vi "digital_demod_host_sp_step.vi"() -> ()   [LabVIEW 2018]
uses:
  <vilib>/userdefined/High Color/nirio_resource_hc.ctl
  <vilib>/LabVIEW Targets/FPGA/RIO/nirio_PxiTriggers.ctl
  <vilib>/UPVI/lvhdf5/file.llb/LVH5F Operation.ctl
  <vilib>/UPVI/lvhdf5/dataset.llb/LVH5D Operation.ctl
  <vilib>/Utility/miscctls.llb/LVRectTypeDef.ctl
  <vilib>/UPVI/lvhdf5/group.llb/H5G_obj_t.ctl
  <vilib>/FPGAPlugInAG/PXI-7854R/niLvFpga_Open_PXI-7854R.vi
  <vilib>/rvi/interface/common/dynamic/niFpgaDynamicAddResources.vi
  <vilib>/FPGAPlugInAG/Dynamic/niLvFpga_Run_Dynamic.vi
  <vilib>/LabVIEW Targets/FPGA/RIO/nirioReserveTrigger.vi
  <vilib>/Utility/error.llb/Error Cluster From Error Code.vi
  <vilib>/rvi/errors/niLvFpgaAdjustHostInterfaceError.vi
  <vilib>/UPVI/lvhdf5/utility.llb/Select HDF5 Dialog.vi
  <vilib>/UPVI/lvhdf5/utility.llb/Select HDF5 Dialog (Object Only).vi
  <vilib>/UPVI/lvhdf5/dataset.llb/Simple H5Dwrite (Variant).vi
  <vilib>/FPGAPlugInAG/Dynamic/niLvFpga_Close_Dynamic.vi
  <vilib>/rvi/interface/nirviOpenFPGA/nirviOpenFPGA.xnode
  FPGA Bitfiles/digitaldemod_FPGATarget_digitaldemodfpga_GFAocKRMO-I.lvbitx
  <vilib>/rvi/interface/nirviMethod/nirviMethod.xnode
  <vilib>/rvi/interface/nirviReadWriteControl/nirviReadWriteControl.xnode
  <vilib>/UPVI/lvhdf5/dataset.llb/Simple H5Dwrite.xnode
  <vilib>/UPVI/lvhdf5/library.llb/HDF5 Ref.ctl
  <vilib>/rvi/interface/nirviCloseFPGA/nirviCloseFPGA.xnode
  <vilib>/rvi/interface/Simulation/niFpgaSimulationCallBeginRW.vi
  <vilib>/rvi/errors/niLvFpgaMergeErrorWithErrorCode.vi
  <vilib>/FPGAPlugInAG/Dynamic/niLvFpga_ReadFifo_Dynamic.vi
  NiFpgaLv.dll
  <vilib>/FPGAPlugInAG/Dynamic/niLvFpga_StartFifo_Dynamic.vi
  <vilib>/FPGAPlugInAG/Dynamic/niLvFpga_StopFifo_Dynamic.vi
  FPGA Timekeeper 1.1b0/FPGA Timekeeper.lvlib
  <vilib>/UPVI/lvhdf5/identifier.llb/Not an HDF5 Refnum Constant.vi
  <vilib>/UPVI/lvhdf5/dataset.llb/OpenCreateReplace Dataset by Element Type.vi
  <vilib>/UPVI/lvhdf5/dataspace.llb/H5Sselect_hyperslab.vi
  <vilib>/UPVI/lvhdf5/dataset.llb/H5Dwrite (Variant).vi
  <vilib>/UPVI/lvhdf5/dataset.llb/H5Dget_space.vi
  <vilib>/UPVI/lvhdf5/attribute.llb/private/LVH5AwriteWDTAttrs.vi
  <vilib>/UPVI/lvhdf5/dataspace.llb/H5Sclose.vi
  <vilib>/UPVI/lvhdf5/dataset.llb/H5Dclose.vi
  <vilib>/UPVI/lvhdf5/utility.llb/Select HDF5 Dialog (File and Object).vi
panel:
  in  "subtract_zfb_ndelay":u8=1
  in  "subtract_zfb_delay":bool=TRUE
  out "pow_fb":i16(graph)=-2000
  in  "subtract_zfb_i_scale":fxp<+/-,32,16>=-17.0
  in  "subtract_zfb_p_scale":fxp<+/-,32,16>=-23.0
  in  "subtract_zfb_d_scale":fxp<+/-,32,16>=-13.0
  in  "subtract_zfb_from_powerr":bool=TRUE
  in  "sum_z-pow_fb":bool=TRUE
  in  "delta_pow_set_llim":fxp<+/-,32,32>=-80000.0
  in  "delta_pow_set_ulim":fxp<+/-,32,32>=80000.0
  in  "fb_on_powset":bool
  in  "pow_lower_lim":i16=-2000
  in  "pow_upper_lim":i16=2000
  in  "pow_dc_offset":i16=-16000
  in  "pow_dg":fxp<+/-,32,16>
  in  "pow_pg":fxp<+/-,32,16>
  in  "pow_fb":bool=TRUE
  out "pow_set_actual":fxp<+/-,33,33>=-165000.0
  in  "reset_pow_accum":bool
  in  "pow_bitshift":i16=-6
  in  "pow_fb_bitshift":i16=-16
  in  "pow_ig":fxp<+/-,32,16>=0.001495361328125
  in  "pow_set_user":fxp<+/-,32,32>=-165000.0
  out "pow":i32(graph)=-95038
  out "delta_pow_set":dbl(graph)
  in  "DAQ_trig":bool
  in  "save_data":bool=TRUE
  out "z_fb_tot":i16(graph)=-20670
  in  "z_off_restart":bool
  in  "z_off_step":i16=-17500
  in  "z_off_start":i16=-17500
  in  "step_z_offset":bool
  in  "z_set_step":fxp<+/-,32,32>
  in  "step_z_set":bool
  out "z_set_user":fxp<+/-,32,32>
  in  "set_z_init":bool
  in  "reset_zphi_and_change":bool
  in  "reset_z_accum":bool
  in  "z_lower_lim":i16=-3000
  in  "z_upper_lim":i16=3000
  in  "z_fb_bitshift":i16=-16
  in  "z_ig":fxp<+/-,32,16>=-1.52587890625e-05
  in  "z_dg":fxp<+/-,32,16>=-0.100006103515625
  in  "z_pg":fxp<+/-,32,16>=-0.0200042724609375
  in  "z_bitshift":i16
  in  "z_set_init":fxp<+/-,32,32>
  in  "z_dc_offset":i16
  in  "z_internal_inject_scale":i16=400
  in  "z_internal_inject_freq":fxp<+,32,0>=2.00001522898674e-05 format="%#_32g"
  in  "add_sin":bool
  in  "show_quad":bool=TRUE
  out "delta_phi":cluster{dbl, dbl, dbl, dbl}(graph)={0.0, -13274.154479980469, -0.0958251953125, -57742.00476074219}
  in  "xy2_bitshift":i16
  in  "xy_fb_bitshift":i16=-16
  in  "y_lower_lim":i16=-1000
  in  "y_upper_lim":i16=1000
  in  "y_dg":fxp<+/-,32,16>=-0.0050048828125
  in  "x_lower_lim":i16=-1000
  in  "x_upper_lim":i16=1000
  in  "x_dg":fxp<+/-,32,16>=0.0050048828125
  in  "xy_bitshift":i16=-10
  in  "y_dc_offset":i16
  in  "x_dc_offset":i16
  in  "downsample->xyz":bool
  in  "inject_sigs":bool
  in  "Load last pars":bool
  out "config_trig":bool
  in  "block_hardware_trigs":bool
  out "config_loaded":bool
  out "Nsamp_config":u32=100000
  out "fpga_dat_path":path=path "D:/data/20201106/bead1/discharge/fine/turbombar_powfb_xyzcool_elec3_4000mV41Hz0mVdc_113_fpga.h5"
  in  "reset_trigs":bool
  in  "accept_trigs":bool=TRUE
  out "amp4":dbl(graph)=1195.7528991699219
  out "phi4":dbl(graph)=-7818.824462890625
  in  "Change Pars 2":bool
  out "z_fb":i16(graph)=-2670
  out "z":i32(graph)=-100000803
  out "y_fb":i16(graph)=-99
  out "y":i32(graph)=-476679
  out "x_fb":i16(graph)=-48
  out "x":i32(graph)=-117629
  out "Host time (ns)":u64=1605214259796328960
  out "Target time (ns)":u64=1605214259796293720
  in  "downsamp_num":i16=100
  in  "Reset Phi Params":T1={"All Phi?"=FALSE, "Which?"=enum."1"}
  out "amp2":dbl(graph)=13832.032684326172
  out "amp3":dbl(graph)=20215.12060546875
  out "amp0":dbl(graph)=9116.836563110352
  out "amp1":dbl(graph)=20779.648162841797
  out "phi2":dbl(graph)=-204.17840576171875
  out "phi3":dbl(graph)=-57946.087341308594
  in  "subtract_mean":bool=TRUE
  out "loop time":fxp<+,32,32>=2.0
  in  "Change Pars":bool
  out "phi0":dbl(graph)=-204.08258056640625
  out "phi1":dbl(graph)=-13478.237060546875
  in  "counter offset":u32
  in  "phase discont_neg":fxp<+/-,24,12>=-1.0
  in  "phase discont_pos":fxp<+/-,24,12>=1.0
  in  "Reset Phi":bool
  in  "loop timer (usec)":u32=2
  in  "Update ADC Clock":bool
  in  "Host Update Rate (msec)":dbl=1.0 format="%#_13g"
  in  "RIO Device":T2="RIO0"
  # "QPD AMPLITUDES"
  # "QPD PHASES"
  # "BACKSCATTER"
  # "BEAD XYZ + FB"
  # "FEEDBACK NESTING"
  # "POWER FEEDBACK"
  # "Z FEEDBACK"
  # "X FEEDBACK"
  # "Y FEEDBACK"
types:
  T1 = cluster{"All Phi?":bool, "Which?":enum16{"0", "1", "2", "3", "4"}}
  T2 = typedef "nirio_resource_hc.ctl" = tag
  T3 = typedef "nirio_PxiTriggers.ctl" = u16
  T4 = cluster{"phase discont_pos":fxp<+/-,24,12>, "phase discont_neg":fxp<+/-,24,12>, "counter offset":u32, "subtract_mean":bool, "downsamp_num":i16, "xy_bitshift":i16, "x_dg":fxp<+/-,32,16>, "x_upper_lim":i16, "x_lower_lim":i16, "x_dc_offset":i16, "y_dg":fxp<+/-,32,16>, "y_upper_lim":i16, "y_lower_lim":i16, "y_dc_offset":i16, "xy_fb_bitshift":i16, "z_bitshift":i16, "z_set_init":fxp<+/-,32,32>, "z_pg":fxp<+/-,32,16>, "z_dg":fxp<+/-,32,16>, "z_ig":fxp<+/-,32,16>, "z_fb_bitshift":i16, "z_upper_lim":i16, "z_lower_lim":i16, "z_off_start":i16, "inject_sigs":bool, "downsample->xyz":bool, "xy2_bitshift":i16, "add_sin":bool, "z_internal_inject_freq":fxp<+,32,0>, "z_internal_inject_scale":i16, "pow_bitshift":i16, "pow_set_user":fxp<+/-,32,32>, "pow_pg":fxp<+/-,32,16>, "pow_dg":fxp<+/-,32,16>, "pow_ig":fxp<+/-,32,16>, "pow_dc_offset":i16, "pow_upper_lim":i16, "pow_lower_lim":i16, "pow_fb_bitshift":i16, "pow_fb":bool, "fb_on_powset":bool, "delta_pow_set_ulim":fxp<+/-,32,32>, "delta_pow_set_llim":fxp<+/-,32,32>, "sum_z-pow_fb":bool, "subtract_zfb_from_powerr":bool, "subtract_zfb_p_scale":fxp<+/-,32,16>, "subtract_zfb_i_scale":fxp<+/-,32,16>, "subtract_zfb_d_scale":fxp<+/-,32,16>, "subtract_zfb_delay":bool, "subtract_zfb_ndelay":u8}
  T5 = enum16{"open", "replace", "create", "open or create", "replace or create", "replace or create with confirmation"}
  T6 = typedef "LVH5F Operation.ctl" = enum16{"open", "open or create", "create or replace", "create or replace (with confirmation)", "create", "open (read only)"}
  T7 = typedef "LVRectTypeDef.ctl" = cluster{"Left":i16, "Top":i16, "Right":i16, "Bottom":i16}
  T8 = cluster{"Behavior":enum32{"Invalid", "Default", "Floating", "Floating/Auto-Hide", "Modal"}, "Position":T7, "Center":bool, "Title":string}
  T9 = typedef "LVH5D Operation.ctl" = enum16{"open", "replace", "create", "open or create", "create or replace", "create or replace with confirmation"}
  T10 = typedef "H5G_obj_t.ctl" = i32
  T11 = cluster{"Object Types (any)":T10[], "Object Pattern":string}
  T12 = typedef "HDF5 Ref.ctl" = refnum<k1>
  T13 = cluster{fxp<+/-,33,19>, fxp<+/-,33,19>, fxp<+/-,33,19>, fxp<+/-,33,19>}
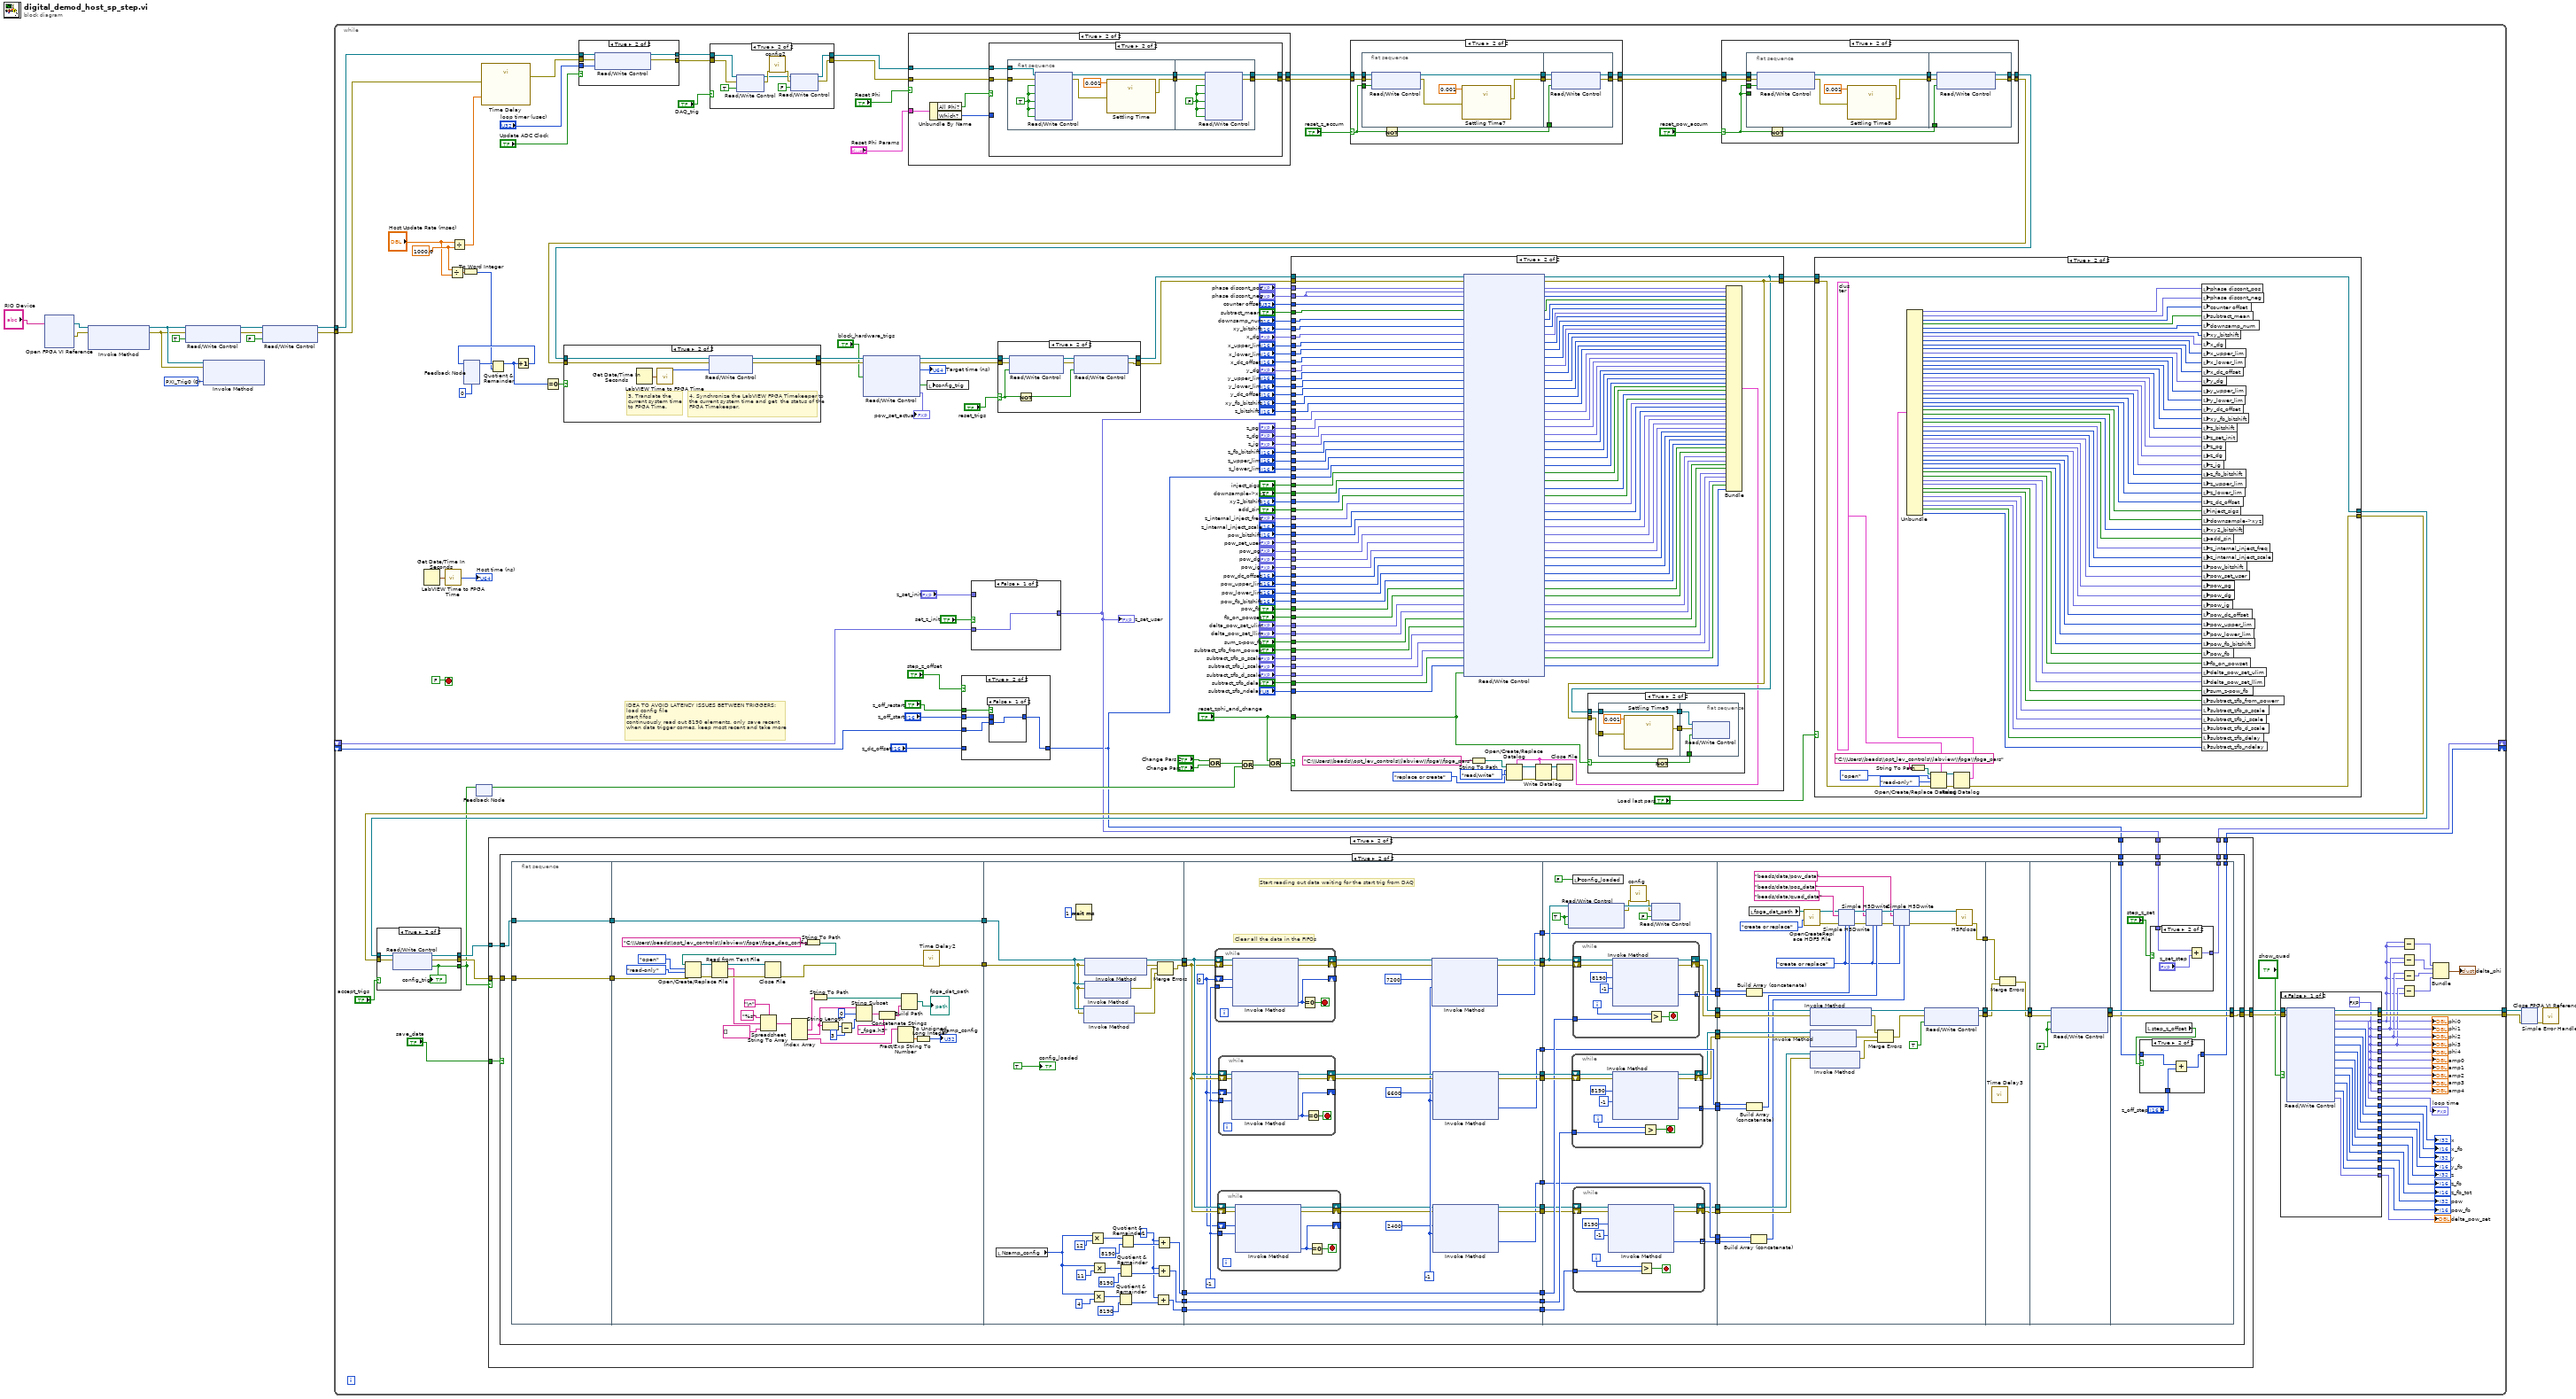
[diagram p0: block diagram]
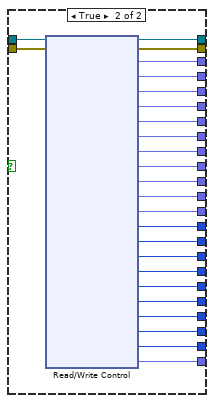
[diagram p7: hidden frame]
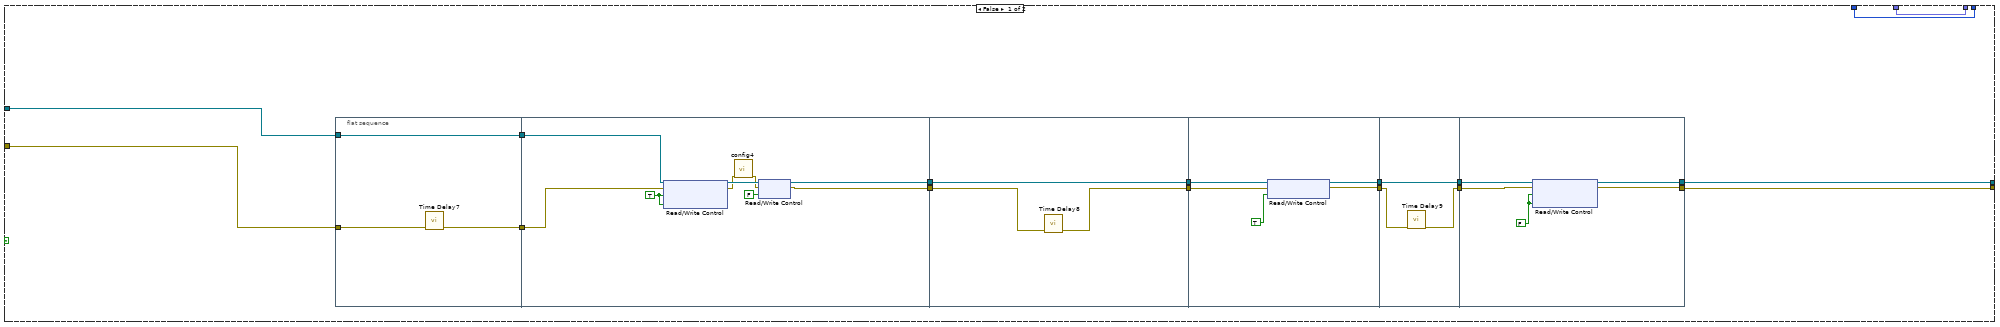
[diagram p12: hidden frame]
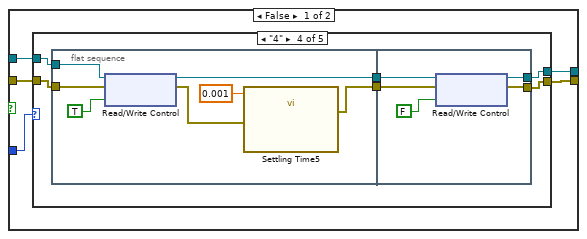
[diagram p20: hidden frame]
diagram:
  w1 = T3 0 items=["PXI_Trig0", "PXI_Trig1", "PXI_Trig2", "PXI_Trig3", "PXI_Trig4", "PXI_Trig5", "PXI_Trig6", "PXI_Trig7"] ("Trigger")
  n1 = xnode "Open FPGA VI Reference"("resource name"="RIO Device") -> ("FPGA VI Reference Out"=w11:refnum<k20>, "error out"=w10:errorcluster)  [unwired: 1 in]
  n2 = xnode "Invoke Method"("FPGA VI Reference In"=w11, "error in"=w10) -> ("FPGA VI Reference Out"=w3:refnum<k20>, "error out"=w2:errorcluster)  [unwired: 1 in]
  n3 = xnode "Read/Write Control"("FPGA VI Reference In"=w3, "error in"=w2, "reset_config_trig"=TRUE ("reset_trig")) -> ("FPGA VI Reference Out"=w6:refnum<k20>, "error out"=w4:errorcluster)
  n4 = xnode "Invoke Method"("FPGA VI Reference In"=w3, "error in"=w2, "Trigger"=w1) -> ()  [unwired: 2 out]
  n5 = xnode "Read/Write Control"("FPGA VI Reference In"=w6, "error in"=w4, "reset_config_trig"=FALSE ("manual_trig")) -> ("FPGA VI Reference Out"=w9:refnum<k20>, "error out"=w8:errorcluster)
  n6 = while {
    tunnel: w8 -> [w166]
    tunnel: w9 -> [w92]
    tunnel: [w159] -> w14
    tunnel: [w158] -> w13
    shift-right: [w70] -> _
    shift-left: _ -> [w71]
    shift-right: [w62] -> _
    shift-left: _ -> [w61]
    stop <- FALSE stop-if-true
    w149 = 1000.0
    # "IDEA TO AVOID LATENCY ISSUES BETWEEN TRIGGERS:\nload config file\nstart fifos\ncontinuously read out 8190 elements, only save recent\nwhen data trigger comes, keep most recent and take more"
    n7 = Get Date/Time In Seconds() -> (seconds since 1Jan1904=w138:timestamp)
    n8 = call "LabVIEW Time to FPGA Time.vi"("LabVIEW time"=w138) -> ("FPGA time (ns)"=→"Host time (ns)":u64)
    n9 = Divide(x=w149, y="Host Update Rate (msec)") -> (x/y=w147:dbl)
    n10 = Divide(x="Host Update Rate (msec)", y=w149) -> (x/y=w167:dbl)
    n11 = To Word Integer(number=w147) -> (16bit integer=w141:i16)
    n12 = feedback #1(i16 0) -> (w143:i16)
    n13 = feedback #2() -> (w73:bool)  [unwired: 1 in]
    n14 = call "Time Delay"("error in (no error)"=w166, "Delay Time (s)"=w167) -> ("error out"=w164:errorcluster)  [unwired: 9 in]
    n15 = Quotient & Remainder(x=w143, y=w141) -> (x-y*floor(x/y)=w140:i16)  [unwired: 1 out]
    n16 = Increment(x=w140) -> (x+1=w142:i16)
    n17 = feedback-in #1(w142) -> ()
    n18 = Equal To 0?(x=w140) -> (x = 0?=w145:bool)
    n19 = case shown="True" "Update ADC Clock" {
      tunnel: w92 -> [w1505 w1510]
      tunnel: w164 -> [w1504 w1509]
      tunnel: [w1505 w1508] -> w50
      tunnel: [w1504 w1507] -> w49
      tunnel: "loop timer (usec)" -> [_ w1506]
      frame False {
      }
      frame True {
        n20 = xnode "Read/Write Control"("FPGA VI Reference In"=w1510, "error in"=w1509, "loop timer (usec)"=w1506) -> ("FPGA VI Reference Out"=w1508:refnum<k20>, "error out"=w1507:errorcluster)
      }
    }
    n21 = case shown="True" "DAQ_trig" {
      tunnel: w50 -> [w191 w195]
      tunnel: w49 -> [w190 w194]
      tunnel: [w191 w193] -> w48
      tunnel: [w190 w192] -> w47
      frame False {
      }
      frame True {
        n22 = xnode "Read/Write Control"("FPGA VI Reference In"=w195, "error in"=w194, "TRIG0"=TRUE) -> ("FPGA VI Reference Out"=w197:refnum<k20>, "error out"=w198:errorcluster)
        n23 = call "config2"("error in (no error)"=w198) -> ("error out"=w199:errorcluster)  [unwired: 10 in]
        n24 = xnode "Read/Write Control"("FPGA VI Reference In"=w197, "error in"=w199, "TRIG0"=FALSE) -> ("FPGA VI Reference Out"=w193:refnum<k20>, "error out"=w192:errorcluster)
      }
    }
    n25 = case shown="True" "Reset Phi" {
      tunnel: w48 -> [w1383 w1390]
      tunnel: w47 -> [w1382 w1389]
      tunnel: [w1383 w1387] -> w96
      tunnel: [w1382 w1388] -> w95
      tunnel: "Reset Phi Params" -> [_ w1386]
      frame False {
      }
      frame True {
        n26 = Unbundle By Name(w1386) -> ("All Phi?"=w1385:bool, "Which?"=w1384:enum16{"0", "1", "2", "3", "4"})
        n27 = case shown="True" w1385 {
          tunnel: w1390 -> [w1395 w1489]
          tunnel: w1389 -> [w1394 w1488]
          tunnel: [w1392 w1487] -> w1388
          tunnel: [w1393 w1486] -> w1387
          tunnel: w1384 -> [w1391 _]
          frame False {
            n28 = case shown="\"4\"" w1391 {
              tunnel: w1395 -> [w1399 w1417 w1435 w1453 w1471]
              tunnel: w1394 -> [w1398 w1416 w1434 w1452 w1470]
              tunnel: [w1397 w1415 w1433 w1451 w1469] -> w1393
              tunnel: [w1396 w1414 w1432 w1450 w1468] -> w1392
              frame "1" {
                n29 = flat-sequence {
                  tunnel: w1399 -> [w1408]
                  tunnel: w1398 -> [w1407]
                  tunnel: [w1406] -> w1401
                  tunnel: [w1403] -> w1400
                  tunnel: w1401 -> [w1413]
                  tunnel: w1400 -> [w1412]
                  tunnel: [w1411] -> w1397
                  tunnel: [w1410] -> w1396
                  frame #0 {
                    n30 = xnode "Read/Write Control"("FPGA VI Reference In"=w1408, "error in"=w1407, "reset_phi1"=TRUE) -> ("FPGA VI Reference Out"=w1406:refnum<k20>, "error out"=w1404:errorcluster)
                    n31 = call "Settling Time2"("error in (no error)"=w1404, "Delay Time (s)"=0.001) -> ("error out"=w1403:errorcluster)  [unwired: 9 in]
                  }
                  frame #1 {
                    n32 = xnode "Read/Write Control"("FPGA VI Reference In"=w1413, "error in"=w1412, "reset_phi1"=FALSE) -> ("FPGA VI Reference Out"=w1411:refnum<k20>, "error out"=w1410:errorcluster)
                  }
                }
              }
              frame "2" {
                n33 = flat-sequence {
                  tunnel: w1417 -> [w1426]
                  tunnel: w1416 -> [w1425]
                  tunnel: [w1424] -> w1419
                  tunnel: [w1421] -> w1418
                  tunnel: w1419 -> [w1431]
                  tunnel: w1418 -> [w1430]
                  tunnel: [w1429] -> w1415
                  tunnel: [w1428] -> w1414
                  frame #0 {
                    n34 = xnode "Read/Write Control"("FPGA VI Reference In"=w1426, "error in"=w1425, "reset_phi2"=TRUE) -> ("FPGA VI Reference Out"=w1424:refnum<k20>, "error out"=w1422:errorcluster)
                    n35 = call "Settling Time3"("error in (no error)"=w1422, "Delay Time (s)"=0.001) -> ("error out"=w1421:errorcluster)  [unwired: 9 in]
                  }
                  frame #1 {
                    n36 = xnode "Read/Write Control"("FPGA VI Reference In"=w1431, "error in"=w1430, "reset_phi2"=FALSE) -> ("FPGA VI Reference Out"=w1429:refnum<k20>, "error out"=w1428:errorcluster)
                  }
                }
              }
              frame "3" {
                n37 = flat-sequence {
                  tunnel: w1435 -> [w1444]
                  tunnel: w1434 -> [w1443]
                  tunnel: [w1442] -> w1437
                  tunnel: [w1439] -> w1436
                  tunnel: w1437 -> [w1449]
                  tunnel: w1436 -> [w1448]
                  tunnel: [w1447] -> w1433
                  tunnel: [w1446] -> w1432
                  frame #0 {
                    n38 = xnode "Read/Write Control"("FPGA VI Reference In"=w1444, "error in"=w1443, "reset_phi3"=TRUE) -> ("FPGA VI Reference Out"=w1442:refnum<k20>, "error out"=w1440:errorcluster)
                    n39 = call "Settling Time4"("error in (no error)"=w1440, "Delay Time (s)"=0.001) -> ("error out"=w1439:errorcluster)  [unwired: 9 in]
                  }
                  frame #1 {
                    n40 = xnode "Read/Write Control"("FPGA VI Reference In"=w1449, "error in"=w1448, "reset_phi3"=FALSE) -> ("FPGA VI Reference Out"=w1447:refnum<k20>, "error out"=w1446:errorcluster)
                  }
                }
              }
              frame "4" {
                n41 = flat-sequence {
                  tunnel: w1453 -> [w1462]
                  tunnel: w1452 -> [w1461]
                  tunnel: [w1460] -> w1455
                  tunnel: [w1457] -> w1454
                  tunnel: w1455 -> [w1467]
                  tunnel: w1454 -> [w1466]
                  tunnel: [w1465] -> w1451
                  tunnel: [w1464] -> w1450
                  frame #0 {
                    n42 = xnode "Read/Write Control"("FPGA VI Reference In"=w1462, "error in"=w1461, "reset_phi4"=TRUE) -> ("FPGA VI Reference Out"=w1460:refnum<k20>, "error out"=w1458:errorcluster)
                    n43 = call "Settling Time5"("error in (no error)"=w1458, "Delay Time (s)"=0.001) -> ("error out"=w1457:errorcluster)  [unwired: 9 in]
                  }
                  frame #1 {
                    n44 = xnode "Read/Write Control"("FPGA VI Reference In"=w1467, "error in"=w1466, "reset_phi4"=FALSE) -> ("FPGA VI Reference Out"=w1465:refnum<k20>, "error out"=w1464:errorcluster)
                  }
                }
              }
              frame "0" {
                n45 = flat-sequence {
                  tunnel: w1471 -> [w1480]
                  tunnel: w1470 -> [w1479]
                  tunnel: [w1478] -> w1473
                  tunnel: [w1475] -> w1472
                  tunnel: w1473 -> [w1485]
                  tunnel: w1472 -> [w1484]
                  tunnel: [w1483] -> w1469
                  tunnel: [w1482] -> w1468
                  frame #0 {
                    n46 = xnode "Read/Write Control"("FPGA VI Reference In"=w1480, "error in"=w1479, "reset_phi0"=TRUE) -> ("FPGA VI Reference Out"=w1478:refnum<k20>, "error out"=w1476:errorcluster)
                    n47 = call "Settling Time6"("error in (no error)"=w1476, "Delay Time (s)"=0.001) -> ("error out"=w1475:errorcluster)  [unwired: 9 in]
                  }
                  frame #1 {
                    n48 = xnode "Read/Write Control"("FPGA VI Reference In"=w1485, "error in"=w1484, "reset_phi0"=FALSE) -> ("FPGA VI Reference Out"=w1483:refnum<k20>, "error out"=w1482:errorcluster)
                  }
                }
              }
            }
          }
          frame True {
            n49 = flat-sequence {
              tunnel: w1489 -> [w1498]
              tunnel: w1488 -> [w1497]
              tunnel: [w1496] -> w1491
              tunnel: [w1493] -> w1490
              tunnel: w1491 -> [w1503]
              tunnel: w1490 -> [w1502]
              tunnel: [w1501] -> w1486
              tunnel: [w1500] -> w1487
              frame #0 {
                w1492 = TRUE
                n50 = xnode "Read/Write Control"("FPGA VI Reference In"=w1498, "error in"=w1497, "reset_phi0"=w1492, "reset_phi1"=w1492, "reset_phi2"=w1492, "reset_phi3"=w1492, "reset_phi4"=w1492) -> ("FPGA VI Reference Out"=w1496:refnum<k20>, "error out"=w1494:errorcluster)
                n51 = call "Settling Time"("error in (no error)"=w1494, "Delay Time (s)"=0.001) -> ("error out"=w1493:errorcluster)  [unwired: 9 in]
              }
              frame #1 {
                w1499 = FALSE
                n52 = xnode "Read/Write Control"("FPGA VI Reference In"=w1503, "error in"=w1502, "reset_phi0"=w1499, "reset_phi1"=w1499, "reset_phi2"=w1499, "reset_phi3"=w1499, "reset_phi4"=w1499) -> ("FPGA VI Reference Out"=w1501:refnum<k20>, "error out"=w1500:errorcluster)
              }
            }
          }
        }
      }
    }
    n53 = case shown="True" "step_z_offset" {
      tunnel: [w201 w202] -> w63
      tunnel: "z_dc_offset" -> [w201 _]
      tunnel: w61 -> [_ w204]
      tunnel: "z_off_start" -> [_ w205]
      tunnel: "z_off_restart" -> [_ w203]
      frame False {
      }
      frame True {
        n54 = case shown="False" w203 {
          tunnel: w205 -> [_ w207]
          tunnel: w204 -> [w206 _]
          tunnel: [w206 w207] -> w202
          frame False {
          }
          frame True {
          }
        }
      }
    }
    n55 = case shown="False" "set_z_init" {
      tunnel: [w208 w209] -> w69
      tunnel: "z_set_init" -> [_ w209]
      tunnel: w71 -> [w208 _]
      frame False {
      }
      frame True {
      }
    }
    "z_set_user" <- w69
    n56 = Or(x="Change Pars 2", y="Change Pars") -> (x .or. y?=w24:bool)
    n57 = Or(x=w24, y=w73) -> (x .or. y?=w22:bool)
    n58 = Or(x="reset_zphi_and_change", y=w22) -> (x .or. y?=w21:bool)
    n59 = case shown="True" "reset_z_accum" {
      selector: "reset_z_accum" -> [_ w317]
      tunnel: w96 -> [w315 w323]
      tunnel: w95 -> [w314 w322]
      tunnel: [w315 w321] -> w46
      tunnel: [w314 w320] -> w45
      frame False {
      }
      frame True {
        n60 = flat-sequence {
          tunnel: w323 -> [w330]
          tunnel: w322 -> [w329]
          tunnel: w317 -> [w327]
          tunnel: [w328] -> w319
          tunnel: [w324] -> w318
          tunnel: [w332] -> w320
          tunnel: [w333] -> w321
          tunnel: w319 -> [w335]
          tunnel: w318 -> [w334]
          tunnel: w316 -> [w331]
          frame #0 {
            n61 = xnode "Read/Write Control"("FPGA VI Reference In"=w330, "error in"=w329, "reset_z_accum"=w327) -> ("FPGA VI Reference Out"=w328:refnum<k20>, "error out"=w325:errorcluster)
            n62 = call "Settling Time7"("error in (no error)"=w325, "Delay Time (s)"=0.001) -> ("error out"=w324:errorcluster)  [unwired: 9 in]
          }
          frame #1 {
            n63 = xnode "Read/Write Control"("FPGA VI Reference In"=w335, "error in"=w334, "reset_z_accum"=w331) -> ("FPGA VI Reference Out"=w333:refnum<k20>, "error out"=w332:errorcluster)
          }
        }
        n64 = Not(x=w317) -> (.not. x?=w316:bool)
      }
    }
    n65 = case shown="True" "reset_pow_accum" {
      selector: "reset_pow_accum" -> [_ w172]
      tunnel: w46 -> [w169 w174]
      tunnel: w45 -> [w168 w173]
      tunnel: [w169 w171] -> w43
      tunnel: [w168 w170] -> w42
      frame False {
      }
      frame True {
        n66 = flat-sequence {
          tunnel: w174 -> [w184]
          tunnel: w173 -> [w183]
          tunnel: w172 -> [w181]
          tunnel: [w182] -> w177
          tunnel: [w178] -> w176
          tunnel: w172 -> [_]
          tunnel: [w185] -> _
          tunnel: [w187] -> w171
          tunnel: w177 -> [w189]
          tunnel: w176 -> [w188]
          tunnel: w175 -> [w186]
          tunnel: [w185] -> w170
          frame #0 {
            n67 = xnode "Read/Write Control"("FPGA VI Reference In"=w184, "error in"=w183, "reset_pow_accum"=w181) -> ("FPGA VI Reference Out"=w182:refnum<k20>, "error out"=w179:errorcluster)
            n68 = call "Settling Time8"("error in (no error)"=w179, "Delay Time (s)"=0.001) -> ("error out"=w178:errorcluster)  [unwired: 9 in]
          }
          frame #1 {
            n69 = xnode "Read/Write Control"("FPGA VI Reference In"=w189, "error in"=w188, "reset_pow_accum"=w186) -> ("FPGA VI Reference Out"=w187:refnum<k20>, "error out"=w185:errorcluster)
          }
        }
        n70 = Not(x=w172) -> (.not. x?=w175:bool)
      }
    }
    n71 = case shown="True" w145 {
      tunnel: w42 -> [w1295 w1300]
      tunnel: w43 -> [w1296 w1299]
      tunnel: [w1296 w1298] -> w136
      tunnel: [w1295 w1297] -> w135
      frame False {
      }
      frame True {
        # "4. Synchronize the LabVIEW FPGA Timekeeper to the current system time and get  the status of the FPGA Timekeeper."
        # "3. Translate the current system time to FPGA Time."
        n72 = Get Date/Time In Seconds() -> (seconds since 1Jan1904=w1302:timestamp)
        n73 = call "LabVIEW Time to FPGA Time.vi"("LabVIEW time"=w1302) -> ("FPGA time (ns)"=w1301:u64)
        n74 = xnode "Read/Write Control"("FPGA VI Reference In"=w1299, "error in"=w1300, "RT time (ns)"=w1301) -> ("FPGA VI Reference Out"=w1298:refnum<k20>, "error out"=w1297:errorcluster)
      }
    }
    n75 = xnode "Read/Write Control"("FPGA VI Reference In"=w136, "error in"=w135, "block_config_trig"="block_hardware_trigs") -> ("FPGA VI Reference Out"=w107:refnum<k20>, "error out"=w106:errorcluster, "time (ns)"=→"Target time (ns)":u64, "config_trig"=w93:bool, "pow_set_actual"=→"pow_set_actual":fxp<+/-,33,33>)
    n76 = local write "config_trig"(w93) -> ()
    n77 = case shown="True" "reset_trigs" {
      selector: "reset_trigs" -> [_ w1288]
      tunnel: w107 -> [w1286 w1294]
      tunnel: w106 -> [w1285 w1293]
      tunnel: [w1286 w1290] -> w103
      tunnel: [w1285 w1289] -> w102
      frame False {
      }
      frame True {
        n78 = xnode "Read/Write Control"("FPGA VI Reference In"=w1294, "error in"=w1293, "reset_config_trig"=w1288) -> ("FPGA VI Reference Out"=w1292:refnum<k20>, "error out"=w1291:errorcluster)
        n79 = Not(x=w1288) -> (.not. x?=w1287:bool)
        n80 = xnode "Read/Write Control"("FPGA VI Reference In"=w1292, "error in"=w1291, "reset_config_trig"=w1287) -> ("FPGA VI Reference Out"=w1290:refnum<k20>, "error out"=w1289:errorcluster)
      }
    }
    n81 = case shown="True" w21 {
      tunnel: w102 -> [w1304 w1367]
      tunnel: [w1304 w1310] -> w89
      tunnel: [w1303 w1309] -> w91
      tunnel: w103 -> [w1303 w1368]
      tunnel: "phase discont_pos" -> [_ w1366]
      tunnel: "phase discont_neg" -> [_ w1365]
      tunnel: "counter offset" -> [_ w1364]
      tunnel: "subtract_mean" -> [_ w1363]
      tunnel: "downsamp_num" -> [_ w1362]
      tunnel: "x_dc_offset" -> [_ w1357]
      tunnel: "y_dc_offset" -> [_ w1353]
      tunnel: w63 -> [_ w1343]
      tunnel: w69 -> [_ w1350]
      tunnel: "xy_bitshift" -> [_ w1361]
      tunnel: "x_dg" -> [_ w1360]
      tunnel: "x_upper_lim" -> [_ w1359]
      tunnel: "x_lower_lim" -> [_ w1358]
      tunnel: "y_dg" -> [_ w1356]
      tunnel: "y_upper_lim" -> [_ w1355]
      tunnel: "y_lower_lim" -> [_ w1354]
      tunnel: "z_bitshift" -> [_ w1351]
      tunnel: "z_pg" -> [_ w1349]
      tunnel: "z_dg" -> [_ w1348]
      tunnel: "z_ig" -> [_ w1347]
      tunnel: "z_fb_bitshift" -> [_ w1346]
      tunnel: "z_upper_lim" -> [_ w1345]
      tunnel: "z_lower_lim" -> [_ w1344]
      tunnel: "xy_fb_bitshift" -> [_ w1352]
      tunnel: "inject_sigs" -> [_ w1334]
      tunnel: "downsample->xyz" -> [_ w1333]
      tunnel: "xy2_bitshift" -> [_ w1332]
      tunnel: "add_sin" -> [_ w1331]
      tunnel: "z_internal_inject_freq" -> [_ w1330]
      tunnel: "z_internal_inject_scale" -> [_ w1329]
      tunnel: "pow_set_user" -> [_ w1327]
      tunnel: "pow_ig" -> [_ w1326]
      tunnel: "pow_fb_bitshift" -> [_ w1320]
      tunnel: "pow_bitshift" -> [_ w1328]
      tunnel: "fb_on_powset" -> [_ w1318]
      tunnel: "delta_pow_set_ulim" -> [_ w1317]
      tunnel: "delta_pow_set_llim" -> [_ w1316]
      tunnel: "pow_fb" -> [_ w1319]
      tunnel: "pow_pg" -> [_ w1324]
      tunnel: "pow_dg" -> [_ w1325]
      tunnel: "pow_dc_offset" -> [_ w1323]
      tunnel: "pow_upper_lim" -> [_ w1322]
      tunnel: "pow_lower_lim" -> [_ w1321]
      tunnel: "sum_z-pow_fb" -> [_ w1315]
      tunnel: "subtract_zfb_from_powerr" -> [_ w1314]
      tunnel: "subtract_zfb_d_scale" -> [_ w1313]
      tunnel: "subtract_zfb_p_scale" -> [_ w1312]
      tunnel: "subtract_zfb_i_scale" -> [_ w1311]
      tunnel: "reset_zphi_and_change" -> [_ w1307]
      tunnel: "subtract_zfb_delay" -> [_ w1306]
      tunnel: "subtract_zfb_ndelay" -> [_ w1305]
      frame False {
      }
      frame True {
        n82 = xnode "Read/Write Control"("FPGA VI Reference In"=w1368, "error in"=w1367, "discont_pos"=w1366, "discont_neg"=w1365, "Counter Offset"=w1364, "subtract_mean"=w1363, "downsamp_num"=w1362, "xy_bitshift"=w1361, "x_dg"=w1360, "x_upper_lim"=w1359, "x_lower_lim"=w1358, "x_dc_offset"=w1357, "y_dg"=w1356, "y_upper_lim"=w1355, "y_lower_lim"=w1354, "y_dc_offset"=w1353, "xy_fb_bitshift"=w1352, "z_bitshift"=w1351, "z_set_user"=w1350, "z_pg"=w1349, "z_dg"=w1348, "z_ig"=w1347, "z_fb_bitshift"=w1346, "z_upper_lim"=w1345, "z_lower_lim"=w1344, "z_dc_offset"=w1343, "inject_sigs"=w1334, "downsample->xyz"=w1333, "xy2_bitshift"=w1332, "add_sin"=w1331, "z_internal_inject_freq"=w1330, "z_internal_inject_scale"=w1329, "pow_bitshift"=w1328, "pow_set_user"=w1327, "pow_pg"=w1324, "pow_dg"=w1325, "pow_ig"=w1326, "pow_dc_offset"=w1323, "pow_upper_lim"=w1322, "pow_lower_lim"=w1321, "pow_fb_bitshift"=w1320, "pow_fb"=w1319, "fb_on_pow_set"=w1318, "delta_pow_set_ulim"=w1317, "delta_pow_set_llim"=w1316, "sum_z-pow_fb"=w1315, "subtract_zfb_from_powerr"=w1314, "subtract_zfb_p_scale"=w1312, "subtract_zfb_i_scale"=w1311, "subtract_zfb_d_scale"=w1313, "subtract_zfb_delay"=w1306, "subtract_zfb_ndelay"=w1305, "reset_phi4"=w1307) -> ("FPGA VI Reference Out"=w1309:refnum<k20>, "error out"=w1310:errorcluster)
        n83 = String To Path(string="C:\\Users\\beads\\opt_lev_controls\\labview\\fpga\\fpga_pars") -> (path=w1336:path)
        n84 = case shown="True" w1307 {
          selector: w1307 -> [_ w1370]
          tunnel: w1310 -> [_ w1372]
          tunnel: w1309 -> [_ w1373]
          frame False {
          }
          frame True {
            n85 = flat-sequence {
              tunnel: [w1377] -> w1374
              tunnel: w1373 -> [w1377]
              tunnel: w1372 -> [w1376]
              tunnel: [w1375] -> w1371
              tunnel: w1374 -> [w1381]
              tunnel: w1371 -> [w1380]
              tunnel: w1369 -> [w1379]
              frame #0 {
                n86 = call "Settling Time9"("error in (no error)"=w1376, "Delay Time (s)"=0.001) -> ("error out"=w1375:errorcluster)  [unwired: 9 in]
              }
              frame #1 {
                n87 = xnode "Read/Write Control"("FPGA VI Reference In"=w1381, "error in"=w1380, "reset_phi4"=w1379) -> ()  [unwired: 2 out]
              }
            }
            n88 = Not(x=w1370) -> (.not. x?=w1369:bool)
          }
        }
        n89 = Bundle("phase discont_pos"=w1366, "phase discont_neg"=w1365, "counter offset"=w1364, "subtract_mean"=w1363, "downsamp_num"=w1362, "xy_bitshift"=w1361, "x_dg"=w1360, "x_upper_lim"=w1359, "x_lower_lim"=w1358, "x_dc_offset"=w1357, "y_dg"=w1356, "y_upper_lim"=w1355, "y_lower_lim"=w1354, "y_dc_offset"=w1353, "xy_fb_bitshift"=w1352, "z_bitshift"=w1351, "z_set_init"=w1350, "z_pg"=w1349, "z_dg"=w1348, "z_ig"=w1347, "z_fb_bitshift"=w1346, "z_upper_lim"=w1345, "z_lower_lim"=w1344, "z_off_start"=w1343, "inject_sigs"=w1334, "downsample->xyz"=w1333, "xy2_bitshift"=w1332, "add_sin"=w1331, "z_internal_inject_freq"=w1330, "z_internal_inject_scale"=w1329, "pow_bitshift"=w1328, "pow_set_user"=w1327, "pow_pg"=w1324, "pow_dg"=w1325, "pow_ig"=w1326, "pow_dc_offset"=w1323, "pow_upper_lim"=w1322, "pow_lower_lim"=w1321, "pow_fb_bitshift"=w1320, "pow_fb"=w1319, "fb_on_powset"=w1318, "delta_pow_set_ulim"=w1317, "delta_pow_set_llim"=w1316, "sum_z-pow_fb"=w1315, "subtract_zfb_from_powerr"=w1314, "subtract_zfb_p_scale"=w1312, "subtract_zfb_i_scale"=w1311, "subtract_zfb_d_scale"=w1313, "subtract_zfb_delay"=w1306, "subtract_zfb_ndelay"=w1305) -> (w1308:T4)  [unwired: 1 in]
        n90 = Open/Create/Replace Datalog(5:w1308, 9:enum16{"read/write", "read-only", "write-only"}."read/write" ("access (0:read/write)"), 10:T5."replace or create" ("operation (0:open)"), 11:w1336) -> (0:w1342:errorcluster, 3:w1340:refnum<k1>)  [unwired: 2 in, 1 out]
        n91 = Write Datalog(4:w1342, 6:w1308, 7:w1340) -> (0:w1341:errorcluster, 3:w1339:refnum<k1>)
        n92 = Close File(refnum=w1339, error in=w1341) -> ()  [unwired: 2 out]
      }
    }
    n93 = case shown="True" "Load last pars" {
      tunnel: [w252 w309] -> w90
      tunnel: w91 -> [w252 w309]
      tunnel: [w251 w296] -> w88
      tunnel: w89 -> [w251 w310]
      frame False {
      }
      frame True {
        n94 = String To Path(string="C:\\Users\\beads\\opt_lev_controls\\labview\\fpga\\fpga_pars") -> (path=w313:path)
        n95 = Open/Create/Replace Datalog(5:T4 {"phase discont_pos"=0.0, "phase discont_neg"=0.0, "counter offset"=0, "subtract_mean"=FALSE, "downsamp_num"=0, "xy_bitshift"=0, "x_dg"=0.0, "x_upper_lim"=0, "x_lower_lim"=0, "x_dc_offset"=0, "y_dg"=0.0, "y_upper_lim"=0, "y_lower_lim"=0, "y_dc_offset"=0, "xy_fb_bitshift"=0, "z_bitshift"=0, "z_set_init"=0.0, "z_pg"=0.0, "z_dg"=0.0, "z_ig"=0.0, "z_fb_bitshift"=0, "z_upper_lim"=0, "z_lower_lim"=0, "z_off_start"=0, "inject_sigs"=FALSE, "downsample->xyz"=FALSE, "xy2_bitshift"=0, "add_sin"=FALSE, "z_internal_inject_freq"=0.0, "z_internal_inject_scale"=0, "pow_bitshift"=0, "pow_set_user"=0.0, "pow_pg"=0.0, "pow_dg"=0.0, "pow_ig"=0.0, "pow_dc_offset"=0, "pow_upper_lim"=0, "pow_lower_lim"=0, "pow_fb_bitshift"=0, "pow_fb"=FALSE, "fb_on_powset"=FALSE, "delta_pow_set_ulim"=0.0, "delta_pow_set_llim"=0.0, "sum_z-pow_fb"=FALSE, "subtract_zfb_from_powerr"=FALSE, "subtract_zfb_p_scale"=0.0, "subtract_zfb_i_scale"=0.0, "subtract_zfb_d_scale"=0.0, "subtract_zfb_delay"=FALSE, "subtract_zfb_ndelay"=0} ("output cluster"), 8:w310, 9:enum16{"read/write", "read-only", "write-only"}."read-only" ("access (0:read/write)"), 10:T5."open" ("operation (0:open)"), 11:w313) -> (0:w307:errorcluster, 3:w308:refnum<k1>)  [unwired: 1 in, 1 out]
        n96 = Read Datalog(4:w307, 7:w308) -> (0:w296:errorcluster, 2:w306:T4)  [unwired: 1 in, 1 out]
        n97 = Unbundle(w306) -> ("phase discont_pos"=w305:fxp<+/-,24,12>, "phase discont_neg"=w304:fxp<+/-,24,12>, "counter offset"=w303:u32, "subtract_mean"=w302:bool, "downsamp_num"=w301:i16, "xy_bitshift"=w300:i16, "x_dg"=w299:fxp<+/-,32,16>, "x_upper_lim"=w298:i16, "x_lower_lim"=w297:i16, "x_dc_offset"=w295:i16, "y_dg"=w294:fxp<+/-,32,16>, "y_upper_lim"=w293:i16, "y_lower_lim"=w292:i16, "y_dc_offset"=w291:i16, "xy_fb_bitshift"=w290:i16, "z_bitshift"=w289:i16, "z_set_init"=w288:fxp<+/-,32,32>, "z_pg"=w287:fxp<+/-,32,16>, "z_dg"=w286:fxp<+/-,32,16>, "z_ig"=w285:fxp<+/-,32,16>, "z_fb_bitshift"=w284:i16, "z_upper_lim"=w283:i16, "z_lower_lim"=w282:i16, "z_off_start"=w281:i16, "inject_sigs"=w279:bool, "downsample->xyz"=w278:bool, "xy2_bitshift"=w277:i16, "add_sin"=w276:bool, "z_internal_inject_freq"=w275:fxp<+,32,0>, "z_internal_inject_scale"=w274:i16, "pow_bitshift"=w273:i16, "pow_set_user"=w272:fxp<+/-,32,32>, "pow_pg"=w271:fxp<+/-,32,16>, "pow_dg"=w270:fxp<+/-,32,16>, "pow_ig"=w269:fxp<+/-,32,16>, "pow_dc_offset"=w268:i16, "pow_upper_lim"=w267:i16, "pow_lower_lim"=w266:i16, "pow_fb_bitshift"=w265:i16, "pow_fb"=w264:bool, "fb_on_powset"=w263:bool, "delta_pow_set_ulim"=w262:fxp<+/-,32,32>, "delta_pow_set_llim"=w261:fxp<+/-,32,32>, "sum_z-pow_fb"=w260:bool, "subtract_zfb_from_powerr"=w259:bool, "subtract_zfb_p_scale"=w258:fxp<+/-,32,16>, "subtract_zfb_i_scale"=w257:fxp<+/-,32,16>, "subtract_zfb_d_scale"=w256:fxp<+/-,32,16>, "subtract_zfb_delay"=w254:bool, "subtract_zfb_ndelay"=w253:u8)
        n98 = local write "phase discont_pos"(w305) -> ()
        n99 = local write "phase discont_neg"(w304) -> ()
        n100 = local write "counter offset"(w303) -> ()
        n101 = local write "subtract_mean"(w302) -> ()
        n102 = local write "downsamp_num"(w301) -> ()
        n103 = local write "xy_bitshift"(w300) -> ()
        n104 = local write "x_dg"(w299) -> ()
        n105 = local write "x_upper_lim"(w298) -> ()
        n106 = local write "x_lower_lim"(w297) -> ()
        n107 = local write "x_dc_offset"(w295) -> ()
        n108 = local write "y_dg"(w294) -> ()
        n109 = local write "y_upper_lim"(w293) -> ()
        n110 = local write "y_lower_lim"(w292) -> ()
        n111 = local write "y_dc_offset"(w291) -> ()
        n112 = local write "xy_fb_bitshift"(w290) -> ()
        n113 = local write "z_bitshift"(w289) -> ()
        n114 = local write "z_set_init"(w288) -> ()
        n115 = local write "z_pg"(w287) -> ()
        n116 = local write "z_dg"(w286) -> ()
        n117 = local write "z_ig"(w285) -> ()
        n118 = local write "z_fb_bitshift"(w284) -> ()
        n119 = local write "z_upper_lim"(w283) -> ()
        n120 = local write "z_lower_lim"(w282) -> ()
        n121 = local write "z_dc_offset"(w281) -> ()
        n122 = local write "inject_sigs"(w279) -> ()
        n123 = local write "downsample->xyz"(w278) -> ()
        n124 = local write "xy2_bitshift"(w277) -> ()
        n125 = local write "add_sin"(w276) -> ()
        n126 = local write "z_internal_inject_freq"(w275) -> ()
        n127 = local write "z_internal_inject_scale"(w274) -> ()
        n128 = local write "pow_bitshift"(w273) -> ()
        n129 = local write "pow_set_user"(w272) -> ()
        n130 = local write "pow_pg"(w271) -> ()
        n131 = local write "pow_dg"(w270) -> ()
        n132 = local write "pow_ig"(w269) -> ()
        n133 = local write "pow_dc_offset"(w268) -> ()
        n134 = local write "pow_upper_lim"(w267) -> ()
        n135 = local write "pow_lower_lim"(w266) -> ()
        n136 = local write "pow_fb_bitshift"(w265) -> ()
        n137 = local write "pow_fb"(w264) -> ()
        n138 = local write "fb_on_powset"(w263) -> ()
        n139 = local write "delta_pow_set_ulim"(w262) -> ()
        n140 = local write "delta_pow_set_llim"(w261) -> ()
        n141 = local write "sum_z-pow_fb"(w260) -> ()
        n142 = local write "subtract_zfb_from_powerr"(w259) -> ()
        n143 = local write "subtract_zfb_p_scale"(w258) -> ()
        n144 = local write "subtract_zfb_i_scale"(w257) -> ()
        n145 = local write "subtract_zfb_d_scale"(w256) -> ()
        n146 = local write "subtract_zfb_delay"(w254) -> ()
        n147 = local write "subtract_zfb_ndelay"(w253) -> ()
      }
    }
    n148 = case shown="True" "accept_trigs" {
      selector: "accept_trigs" -> [w338 _]
      tunnel: [w338 w339] -> w57
      tunnel: w88 -> [w336 w343]
      tunnel: w90 -> [w337 w342]
      tunnel: [w337 w341] -> w99
      tunnel: [w336 w340] -> w98
      frame False {
      }
      frame True {
        n149 = xnode "Read/Write Control"("FPGA VI Reference In"=w342, "error in"=w343) -> ("FPGA VI Reference Out"=w341:refnum<k20>, "error out"=w340:errorcluster, "config_trig"=w339:bool)
        "config_trig" <- w339
      }
    }
    n150 = feedback-in #2(w57) -> ()
    n151 = case shown="True" w57 {
      tunnel: w99 -> [w345 w349]
      tunnel: [w345 w356] -> w101
      tunnel: [w344 w355] -> w100
      tunnel: w98 -> [w344 w354]
      tunnel: [w347 w352] -> w70
      tunnel: w69 -> [w347 w353]
      tunnel: w63 -> [w346 w351]
      tunnel: [w346 w350] -> w62
      tunnel: "save_data" -> [_ w348]
      frame False {
      }
      frame True {
        n152 = case shown="True" w348 {
          tunnel: [w359 w418] -> w356
          tunnel: [w360 w417] -> w355
          tunnel: w354 -> [w361 w416]
          tunnel: w353 -> [w358 w415]
          tunnel: [w358 w414] -> w352
          tunnel: w351 -> [w357 w413]
          tunnel: [w357 w412] -> w350
          tunnel: w349 -> [w362 w411]
          frame False {
            n153 = flat-sequence {
              tunnel: [w375] -> w372
              tunnel: w362 -> [w375]
              tunnel: w361 -> [w374]
              tunnel: [w373] -> w371
              tunnel: w372 -> [w379]
              tunnel: w371 -> [w377]
              tunnel: [w378] -> w370
              tunnel: [w376] -> w369
              tunnel: w370 -> [w387]
              tunnel: w369 -> [w386]
              tunnel: [w387] -> w368
              tunnel: [w385] -> w367
              tunnel: w368 -> [w391]
              tunnel: w367 -> [w390]
              tunnel: [w388] -> w366
              tunnel: [w389] -> w365
              tunnel: w366 -> [w395]
              tunnel: w365 -> [w394]
              tunnel: [w395] -> w364
              tunnel: [w393] -> w363
              tunnel: [w396] -> w360
              tunnel: [w397] -> w359
              tunnel: w364 -> [w399]
              tunnel: w363 -> [w398]
              frame #0 {
                n154 = call "Time Delay7"("error in (no error)"=w374) -> ("error out"=w373:errorcluster)  [unwired: 10 in]
              }
              frame #1 {
                w384 = TRUE
                n155 = xnode "Read/Write Control"("FPGA VI Reference In"=w379, "error in"=w377, "block_config_trig"=w384, "TRIG0"=w384) -> ("FPGA VI Reference Out"=w383:refnum<k20>, "error out"=w382:errorcluster)
                n156 = call "config4"("error in (no error)"=w382) -> ("error out"=w381:errorcluster)  [unwired: 10 in]
                n157 = xnode "Read/Write Control"("FPGA VI Reference In"=w383, "error in"=w381, "TRIG0"=FALSE) -> ("FPGA VI Reference Out"=w378:refnum<k20>, "error out"=w376:errorcluster)
              }
              frame #2 {
                n158 = call "Time Delay8"("error in (no error)"=w386) -> ("error out"=w385:errorcluster)  [unwired: 10 in]
              }
              frame #3 {
                n159 = xnode "Read/Write Control"("FPGA VI Reference In"=w391, "error in"=w390, "reset_config_trig"=TRUE) -> ("FPGA VI Reference Out"=w388:refnum<k20>, "error out"=w389:errorcluster)
              }
              frame #4 {
                n160 = call "Time Delay9"("error in (no error)"=w394) -> ("error out"=w393:errorcluster)  [unwired: 10 in]
              }
              frame #5 {
                w400 = FALSE
                n161 = xnode "Read/Write Control"("FPGA VI Reference In"=w399, "error in"=w398, "block_config_trig"=w400, "reset_config_trig"=w400) -> ("FPGA VI Reference Out"=w397:refnum<k20>, "error out"=w396:errorcluster)
              }
            }
          }
          frame True {
            n162 = flat-sequence {
              tunnel: w416 -> [w450]
              tunnel: [w450] -> w448
              tunnel: [w449] -> w447
              tunnel: w411 -> [w449]
              tunnel: [w452] -> w446
              tunnel: w448 -> [w454]
              tunnel: [w451] -> w445
              tunnel: w447 -> [w451]
              tunnel: w446 -> [w483]
              tunnel: [w496] -> w444
              tunnel: [w493] -> w443
              tunnel: [w495] -> w442
              tunnel: [w494] -> w441
              tunnel: w445 -> [w484]
              tunnel: [w485] -> w408
              tunnel: w444 -> [w517]
              tunnel: w443 -> [w518]
              tunnel: [w532] -> w440
              tunnel: [w531] -> w439
              tunnel: [w525] -> w438
              tunnel: [w524] -> w437
              tunnel: [w530] -> w436
              tunnel: w442 -> [w530]
              tunnel: [w529] -> w435
              tunnel: w441 -> [w529]
              tunnel: [w528] -> w434
              tunnel: [w523] -> w433
              tunnel: [w519] -> w409
              tunnel: w408 -> [w519]
              tunnel: [w510] -> w407
              tunnel: [w509] -> w406
              tunnel: [w508] -> w403
              tunnel: w440 -> [w579]
              tunnel: w439 -> [w584]
              tunnel: w438 -> [w583]
              tunnel: w437 -> [w582]
              tunnel: w436 -> [w581]
              tunnel: w435 -> [w580]
              tunnel: [w578] -> w432
              tunnel: w434 -> [w578]
              tunnel: [w577] -> w431
              tunnel: [w576] -> w430
              tunnel: w433 -> [w576]
              tunnel: [w575] -> w429
              tunnel: [w574] -> w428
              tunnel: [w573] -> w427
              tunnel: [w572] -> w426
              tunnel: [w571] -> w425
              tunnel: w409 -> [w562]
              tunnel: w407 -> [w564]
              tunnel: w406 -> [w563]
              tunnel: [w561] -> w405
              tunnel: [w560] -> w404
              tunnel: w403 -> [w560]
              tunnel: [w559] -> w402
              tunnel: [w558] -> w401
              tunnel: w432 -> [w648]
              tunnel: w431 -> [w647]
              tunnel: w430 -> [w646]
              tunnel: w429 -> [w645]
              tunnel: w428 -> [w644]
              tunnel: w427 -> [w643]
              tunnel: w426 -> [w641]
              tunnel: w425 -> [w642]
              tunnel: [w640] -> w424
              tunnel: [w639] -> w423
              tunnel: [w627] -> w410
              tunnel: w405 -> [w620]
              tunnel: w404 -> [w619]
              tunnel: w402 -> [w618]
              tunnel: w401 -> [w617]
              tunnel: w424 -> [w1262]
              tunnel: [w1262] -> w422
              tunnel: w423 -> [w1260]
              tunnel: [w1259] -> w421
              tunnel: w410 -> [w1261]
              tunnel: w422 -> [w1267]
              tunnel: w421 -> [w1266]
              tunnel: [w1265] -> w420
              tunnel: [w1264] -> w419
              tunnel: [w1275] -> w417
              tunnel: [w1276] -> w418
              tunnel: w420 -> [w1276]
              tunnel: w419 -> [w1275]
              tunnel: w415 -> [w1273]
              tunnel: [w1272] -> w414
              tunnel: w413 -> [w1270]
              tunnel: [w1269] -> w412
              frame #0 {
              }
              frame #1 {
                n163 = String To Path(string="C:\\Users\\beads\\opt_lev_controls\\labview\\fpga\\fpga_daq_config") -> (path=w480:path)
                n164 = Open/Create/Replace File(file path (use dialog)=w480, error in=w454, operation (0:open)=T5."open", access (0:read/write)=enum16{"read/write", "read-only", "write-only"}."read-only") -> (refnum out=w477:refnum<file>, error out=w476:errorcluster)  [unwired: 2 in, 1 out]
                n165 = Read from Text File(file (use dialog)=w477, error in=w476) -> (refnum out=w475:refnum<file>, text=w473:string, error out=w474:errorcluster)  [unwired: 2 in, 1 out]
                n166 = Spreadsheet String To Array(delimiter (Tab)="\n", format string="%s", spreadsheet string=w473, array type (2D Dbl)=string[] [] ("array of strings")) -> (array=w469:string[])
                n167 = Close File(refnum=w475, error in=w474) -> (error out=w453:errorcluster)  [unwired: 1 out]
                n168 = Index Array(array=w469) -> (element #1=w468:string, element #2=w465:string, element #3=w457:string)  [unwired: 3 in]
                n169 = String To Path(string=w468) -> (path=w467:path)
                n170 = String Length(string=w465) -> (length=w464:i32)
                n171 = Subtract(x=w464, y=3) -> (x-y=w462:i32)
                n172 = String Subset(string=w465, offset (0)=0, length (rest)=w462) -> (substring=w461:string)
                n173 = Concatenate Strings(w461, "_fpga.h5" ("string")) -> (w459:string)
                n174 = Fract/Exp String To Number(string=w457) -> (number=w456:dbl)  [unwired: 3 in, 1 out]
                n175 = Build Path(base path=w467, name or relative path=w459) -> (appended path=→"fpga_dat_path":path)
                n176 = To Unsigned Long Integer(number=w456) -> (unsigned 32bit integer=→"Nsamp_config":u32)
                n177 = call "Time Delay2"("error in (no error)"=w453) -> ("error out"=w452:errorcluster)  [unwired: 10 in]
              }
              frame #2 {
                w486 = u32 1 ("Extra Samps")
                n178 = local read "Nsamp_config"() -> (w487:u32)
                n179 = Wait (ms)(milliseconds to wait=u32 1) -> ()  [unwired: 1 out]
                n180 = xnode "Invoke Method"("FPGA VI Reference In"=w484, "error in"=w483) -> ("error out"=w482:errorcluster)  [unwired: 1 out]
                n181 = xnode "Invoke Method"("FPGA VI Reference In"=w484, "error in"=w483) -> ("error out"=w498:errorcluster)  [unwired: 1 out]
                n182 = xnode "Invoke Method"("FPGA VI Reference In"=w484, "error in"=w483) -> ("FPGA VI Reference Out"=w493:refnum<k20>, "error out"=w497:errorcluster)
                n183 = Multiply(x=w487, y=u32 12) -> (x*y=w500:u32)
                n184 = Multiply(x=w487, y=u32 4) -> (x*y=w488:u32)
                n185 = Multiply(x=w487, y=u32 11) -> (x*y=w499:u32)
                n186 = Quotient & Remainder(x=w488, y=u32 8190) -> (floor(x/y)=w490:u32)  [unwired: 1 out]
                n187 = Quotient & Remainder(x=w499, y=u32 8190) -> (floor(x/y)=w502:u32)  [unwired: 1 out]
                n188 = Quotient & Remainder(x=w500, y=u32 8190) -> (floor(x/y)=w504:u32)  [unwired: 1 out]
                n189 = Add(x=w486, y=w490) -> (x+y=w485:u32)
                n190 = Add(x=w486, y=w504) -> (x+y=w495:u32)
                n191 = Add(x=w486, y=w502) -> (x+y=w494:u32)
                n192 = Merge Errors(w497, w498, w482) -> (w496:errorcluster)
                "config_loaded" <- TRUE
              }
              frame #3 {
                w514 = -1 ("Timeout (ms)")
                w515 = u32 0 ("Elements Remaining")
                w516 = -1
                # "Start reading out data waiting for the start trig from DAQ"
                # "Clear all the data in the FIFOs"
                n193 = while {
                  tunnel: w516 -> [w552]
                  shift-right: [w554] -> w533
                  shift-left: w518 -> [w557]
                  shift-right: [w553] -> w522
                  shift-left: w517 -> [w556]
                  shift-right: [w551] -> _
                  shift-left: w515 -> [w555]
                  stop <- w550 stop-if-true
                  n194 = xnode "Invoke Method"("FPGA VI Reference In"=w557, "error in"=w556, "Number of Elements"=w555, "Timeout (ms)"=w552) -> ("FPGA VI Reference Out"=w554:refnum<k20>, "error out"=w553:errorcluster, "Elements Remaining"=w551:u32)  [unwired: 1 out]
                  n195 = Equal To 0?(x=w551) -> (x = 0?=w550:bool)
                }
                n196 = while {
                  tunnel: w516 -> [w539]
                  shift-right: [w536] -> _
                  shift-left: w515 -> [w538]
                  shift-right: [w535] -> w513
                  shift-left: w518 -> [w541]
                  shift-right: [w534] -> w512
                  shift-left: w517 -> [w540]
                  stop <- w537 stop-if-true
                  n197 = xnode "Invoke Method"("FPGA VI Reference In"=w541, "error in"=w540, "Number of Elements"=w538, "Timeout (ms)"=w539) -> ("FPGA VI Reference Out"=w535:refnum<k20>, "error out"=w534:errorcluster, "Elements Remaining"=w536:u32)  [unwired: 1 out]
                  n198 = Equal To 0?(x=w536) -> (x = 0?=w537:bool)
                }
                n199 = while {
                  tunnel: w516 -> [w544]
                  shift-right: [w546] -> w527
                  shift-left: w518 -> [w549]
                  shift-right: [w545] -> w526
                  shift-left: w517 -> [w548]
                  shift-right: [w543] -> _
                  shift-left: w515 -> [w547]
                  stop <- w542 stop-if-true
                  n200 = xnode "Invoke Method"("FPGA VI Reference In"=w549, "error in"=w548, "Number of Elements"=w547, "Timeout (ms)"=w544) -> ("FPGA VI Reference Out"=w546:refnum<k20>, "error out"=w545:errorcluster, "Elements Remaining"=w543:u32)  [unwired: 1 out]
                  n201 = Equal To 0?(x=w543) -> (x = 0?=w542:bool)
                }
                n202 = xnode "Invoke Method"("FPGA VI Reference In"=w533, "error in"=w522, "Number of Elements"=u32 7200, "Timeout (ms)"=w514) -> ("FPGA VI Reference Out"=w532:refnum<k20>, "error out"=w531:errorcluster, "Data"=w528:i32[])  [unwired: 1 out]
                n203 = xnode "Invoke Method"("FPGA VI Reference In"=w527, "error in"=w526, "Number of Elements"=u32 6600, "Timeout (ms)"=w514) -> ("FPGA VI Reference Out"=w525:refnum<k20>, "error out"=w524:errorcluster, "Data"=w523:i32[])  [unwired: 1 out]
                n204 = xnode "Invoke Method"("FPGA VI Reference In"=w513, "error in"=w512, "Number of Elements"=u32 2400, "Timeout (ms)"=w514) -> ("FPGA VI Reference Out"=w510:refnum<k20>, "error out"=w509:errorcluster, "Data"=w508:i32[])  [unwired: 1 out]
              }
              frame #4 {
                w569 = TRUE
                n205 = xnode "Read/Write Control"("FPGA VI Reference In"=w579, "block_config_trig"=w569, "TRIG0"=w569) -> ("FPGA VI Reference Out"=w568:refnum<k20>, "error out"=w567:errorcluster)  [unwired: 1 in]
                n206 = while {
                  shift-right: [w600] -> w572
                  shift-left: w583 -> [w604]
                  shift-right: [w599] -> w571
                  shift-left: w582 -> [w603]
                  tunnel: w580 -> [w596]
                  tunnel: [w595] -> w575 mode=concatenating
                  i -> [w598]
                  stop <- w597 stop-if-true
                  n207 = xnode "Invoke Method"("FPGA VI Reference In"=w604, "error in"=w603, "Number of Elements"=u32 8190, "Timeout (ms)"=-1) -> ("FPGA VI Reference Out"=w600:refnum<k20>, "error out"=w599:errorcluster, "Data"=w595:i32[])  [unwired: 1 out]
                  n208 = Greater?(x=w598, y=w596) -> (0:w597:bool)
                }
                n209 = local write "config_loaded"(FALSE) -> ()
                n210 = while {
                  shift-right: [w610] -> w574
                  shift-left: w579 -> [w614]
                  shift-right: [w609] -> w573
                  shift-left: w584 -> [w613]
                  tunnel: w581 -> [w606]
                  tunnel: [w605] -> w577 mode=concatenating
                  i -> [w608]
                  stop <- w607 stop-if-true
                  n211 = xnode "Invoke Method"("FPGA VI Reference In"=w614, "error in"=w613, "Number of Elements"=u32 8190, "Timeout (ms)"=-1) -> ("FPGA VI Reference Out"=w610:refnum<k20>, "error out"=w609:errorcluster, "Data"=w605:i32[])  [unwired: 1 out]
                  n212 = Greater?(x=w608, y=w606) -> (0:w607:bool)
                }
                n213 = while {
                  tunnel: w562 -> [w588]
                  shift-right: [w587] -> w559
                  shift-left: w564 -> [w594]
                  shift-right: [w586] -> w558
                  shift-left: w563 -> [w593]
                  tunnel: [w585] -> w561 mode=concatenating
                  i -> [w590]
                  stop <- w589 stop-if-true
                  n214 = xnode "Invoke Method"("FPGA VI Reference In"=w594, "error in"=w593, "Number of Elements"=u32 8190, "Timeout (ms)"=-1) -> ("FPGA VI Reference Out"=w587:refnum<k20>, "error out"=w586:errorcluster, "Data"=w585:i32[])  [unwired: 1 out]
                  n215 = Greater?(x=w590, y=w588) -> (0:w589:bool)
                }
                n216 = call "config"("error in (no error)"=w567) -> ("error out"=w566:errorcluster)  [unwired: 10 in]
                n217 = xnode "Read/Write Control"("FPGA VI Reference In"=w568, "error in"=w566, "TRIG0"=FALSE) -> ()  [unwired: 2 out]
              }
              frame #5 {
                w621 = LVH5D_Operation."create or replace" ("operation (open or create)")
                n218 = Build Array (concatenate)(w648, w647) -> (w635:i32[])
                n219 = Build Array (concatenate)(w646, w645) -> (w630:i32[])
                n220 = local read "fpga_dat_path"() -> (w637:path)
                n221 = Build Array (concatenate)(w619, w620) -> (w615:i32[])
                n222 = call <vilib>:"OpenCreateReplace HDF5 File.vi"("function (open or create)"=LVH5F_Operation."create or replace", "path"=w637) -> ("error out"=w628:errorcluster, "HDF5 Ref out"=w629:T12)  [unwired: 6 in]
                n223 = xnode "Invoke Method"("FPGA VI Reference In"=w644, "error in"=w643) -> ("FPGA VI Reference Out"=w650:refnum<k20>, "error out"=w652:errorcluster)
                n224 = xnode "Invoke Method"("FPGA VI Reference In"=w641, "error in"=w642) -> ("error out"=w651:errorcluster)  [unwired: 1 out]
                n225 = xnode "Invoke Method"("FPGA VI Reference In"=w618, "error in"=w617) -> ("error out"=w616:errorcluster)  [unwired: 1 out]
                n226 = xnode "Simple H5Dwrite"("Dataset Path"="beads/data/quad_data" ("dataset name"), "error in (no error)"=w628, "operation (open or create)"=w621, "HDF5 Path or Ref"=w629, "Data"=w635) -> ("HDF5 Ref out"=w633:T12, "error out"=w632:errorcluster)  [unwired: 3 in, 1 out]
                n227 = xnode "Simple H5Dwrite"("Dataset Path"="beads/data/pos_data" ("dataset name"), "error in (no error)"=w632, "operation (open or create)"=w621, "HDF5 Path or Ref"=w633, "Data"=w630) -> ("HDF5 Ref out"=w626:T12, "error out"=w625:errorcluster)  [unwired: 3 in, 1 out]
                n228 = Merge Errors(w652, w651, w616) -> (w638:errorcluster)
                n229 = xnode "Simple H5Dwrite"("Dataset Path"="beads/data/pow_data" ("dataset name"), "error in (no error)"=w625, "operation (open or create)"=w621, "HDF5 Path or Ref"=w626, "Data"=w615) -> ("HDF5 Ref out"=w623:T12, "error out"=w624:errorcluster)  [unwired: 3 in, 1 out]
                n230 = xnode "Read/Write Control"("FPGA VI Reference In"=w650, "error in"=w638, "reset_config_trig"=TRUE) -> ("FPGA VI Reference Out"=w640:refnum<k20>, "error out"=w639:errorcluster)
                n231 = call <vilib>:"H5Fclose.vi"("error in (no error)"=w624, "HDF5 Ref"=w623) -> ("error out"=w627:errorcluster)  [unwired: 7 in]
              }
              frame #6 {
                n232 = call "Time Delay3"() -> ()  [unwired: 11 in, 1 out]
                n233 = Merge Errors(w1261, w1260) -> (w1259:errorcluster)
              }
              frame #7 {
                w1263 = FALSE
                n234 = xnode "Read/Write Control"("FPGA VI Reference In"=w1267, "error in"=w1266, "block_config_trig"=w1263, "reset_config_trig"=w1263) -> ("FPGA VI Reference Out"=w1265:refnum<k20>, "error out"=w1264:errorcluster)
              }
              frame #8 {
                n235 = local read "step_z_offset"() -> (w1271:bool)
                n236 = case shown="True" w1271 {
                  tunnel: w1270 -> [w1277 w1280]
                  tunnel: [w1277 w1278] -> w1269
                  tunnel: "z_off_step" -> [_ w1279]
                  frame False {
                  }
                  frame True {
                    n237 = Add(x=w1280, y=w1279) -> (x+y=w1278:i16)
                  }
                }
                n238 = case shown="True" "step_z_set" {
                  tunnel: [w1281 w1283] -> w1272
                  tunnel: w1273 -> [w1281 w1282]
                  frame False {
                  }
                  frame True {
                    n239 = Add(x=w1282, y="z_set_step") -> (x+y=w1283:fxp<+/-,32,32>)
                  }
                }
              }
            }
          }
        }
      }
    }
    n240 = case shown="False" "show_quad" {
      tunnel: [w223 w250] -> w159
      tunnel: [w222 w249] -> w158
      tunnel: [w221 w248] -> w156
      tunnel: [w214 w247] -> w155
      tunnel: [w214 w246] -> w154
      tunnel: [w214 w245] -> w153
      tunnel: [w214 w244] -> w152
      tunnel: [w220 w243] -> w132
      tunnel: [w219 w242] -> w131
      tunnel: [w218 w241] -> w130
      tunnel: [w217 w240] -> w129
      tunnel: [w216 w239] -> w128
      tunnel: [w215 w238] -> w127
      tunnel: [w214 w237] -> w109
      tunnel: [w214 w236] -> w108
      tunnel: w101 -> [w225 w235]
      tunnel: w100 -> [w224 w234]
      tunnel: [w214 w233] -> w83
      tunnel: [w214 w232] -> w82
      tunnel: [w214 w231] -> w81
      tunnel: [w214 w230] -> w80
      tunnel: [w213 w229] -> w58
      tunnel: [w212 w228] -> w37
      tunnel: [w210 w227] -> w19
      tunnel: [w211 w226] -> w18
      frame False {
        w214 = fxp<+/-,32,18> 0.0 ("phi0_full_out")
        n241 = xnode "Read/Write Control"("FPGA VI Reference In"=w225, "error in"=w224) -> ("FPGA VI Reference Out"=w223:refnum<k20>, "error out"=w222:errorcluster, "loop time"=w221:fxp<+,32,32>, "x_shifted"=w220:i32, "x_fb_i16"=w219:i16, "y_shifted"=w218:i32, "y_fb_i16"=w217:i16, "z_shifted"=w216:i32, "z_fb_i16"=w215:i16, "z_fb_tot_i16"=w213:i16, "pow_shifted"=w212:i32, "pow_fb_i16"=w211:i16, "delta_pow_set"=w210:fxp<+/-,32,32>)
      }
      frame True {
        n242 = xnode "Read/Write Control"("FPGA VI Reference In"=w235, "error in"=w234) -> ("FPGA VI Reference Out"=w250:refnum<k20>, "error out"=w249:errorcluster, "phi0_full_out"=w230:fxp<+/-,32,18>, "phi1_full_out"=w233:fxp<+/-,32,18>, "phi2_full_out"=w232:fxp<+/-,32,18>, "phi3_full_out"=w231:fxp<+/-,32,18>, "phi4_full_out"=w237:fxp<+/-,32,18>, "amp0_out"=w244:fxp<+,32,16>, "amp1_out"=w245:fxp<+,32,16>, "amp2_out"=w246:fxp<+,32,16>, "amp3_out"=w247:fxp<+,32,16>, "amp4_out"=w236:fxp<+,32,16>, "loop time"=w248:fxp<+,32,32>, "x_shifted"=w243:i32, "x_fb_i16"=w242:i16, "y_shifted"=w241:i32, "y_fb_i16"=w240:i16, "z_shifted"=w239:i32, "z_fb_i16"=w238:i16, "z_fb_tot_i16"=w229:i16, "pow_shifted"=w228:i32, "pow_fb_i16"=w226:i16, "delta_pow_set"=w227:fxp<+/-,32,32>)
      }
    }
    "phi1" <- w83
    "phi0" <- w80
    "loop time" <- w156
    "phi3" <- w81
    "phi2" <- w82
    "amp1" <- w153
    "amp0" <- w152
    "amp3" <- w155
    "amp2" <- w154
    "x" <- w132
    "x_fb" <- w131
    "y" <- w130
    "y_fb" <- w129
    "z" <- w128
    "z_fb" <- w127
    "phi4" <- w109
    "amp4" <- w108
    "z_fb_tot" <- w58
    "delta_pow_set" <- w19
    "pow" <- w37
    "pow_fb" <- w18
    n243 = Subtract(x=w80, y=w80) -> (x-y=w79:fxp<+/-,33,19>)
    n244 = Subtract(x=w83, y=w80) -> (x-y=w78:fxp<+/-,33,19>)
    n245 = Subtract(x=w82, y=w80) -> (x-y=w77:fxp<+/-,33,19>)
    n246 = Subtract(x=w81, y=w80) -> (x-y=w76:fxp<+/-,33,19>)
    n247 = Bundle(w79, w78, w77, w76) -> (→"delta_phi":T13)  [unwired: 1 in]
  }
  n248 = xnode "Close FPGA VI Reference"("FPGA VI Reference In"=w14, "error in"=w13) -> ("error out"=w15:errorcluster)
  n249 = call <vilib>:"Simple Error Handler.vi"("error in (no error)"=w15) -> ()  [unwired: 4 in, 5 out]
